vi "Lan07.vi"() -> ()   [LabVIEW 2022 SP3]
uses:
  StateMachineControl.ctl
  <vilib>/measure/NI_MAPro.lvlib
  <vilib>/measure/NI_MABase.lvlib
  <vilib>/measure/mascope.llb/Amplitude and Levels 1 chan.vi
panel:
  in  "Amplitude":dbl=1.0 format="%0.2p"
  out "High State Level":dbl format="%.2g"
  out "Pk-Pk Measured":dbl format="%.2p"
  out "Current State":T1
  in  "Stop":bool
  in  "Analyze Data":bool
  in  "Aquire Data":bool
  out "Waveform Graph":waveform(dbl)(graph)
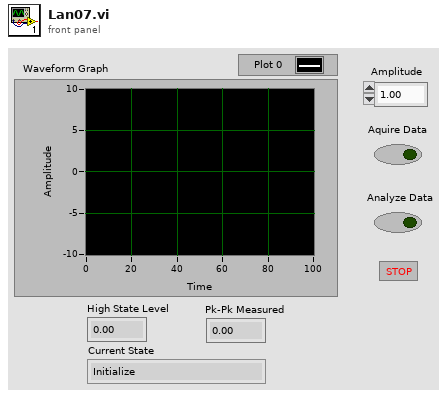
[diagram p1: front panel]
types:
  T1 = typedef "StateMachineControl.ctl" = enum16{"Initialize", "Stop", "Check for UI Events", "Aquire Data", "Analyze Data"}
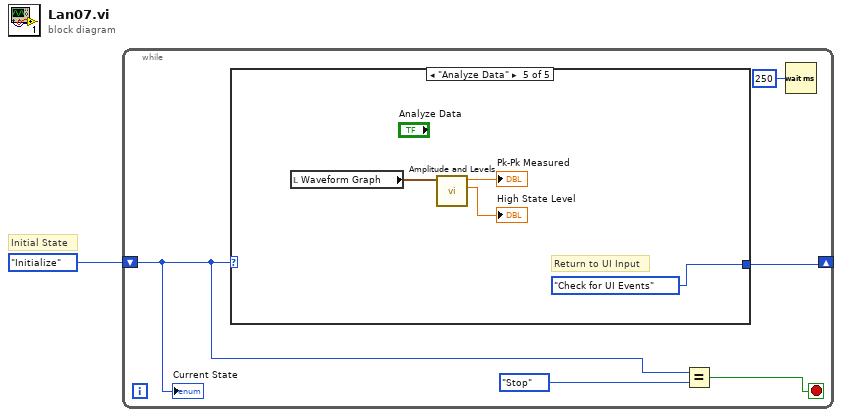
[diagram p0: block diagram]
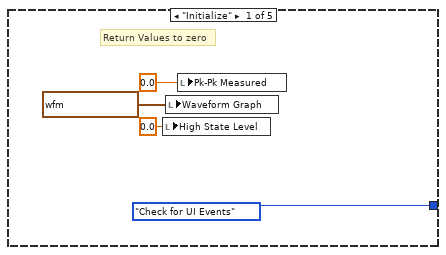
[diagram p2: hidden frame]
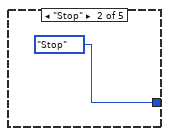
[diagram p3: hidden frame]
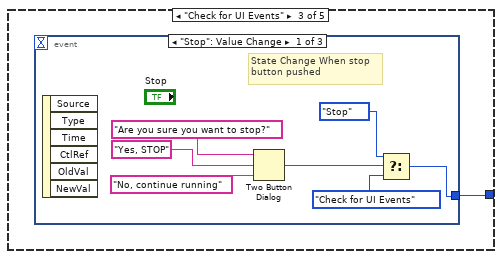
[diagram p4: hidden frame]
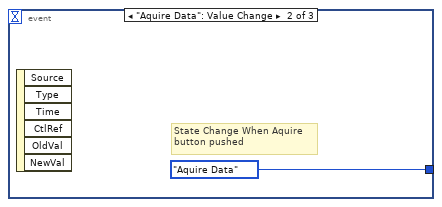
[diagram p5: hidden frame]
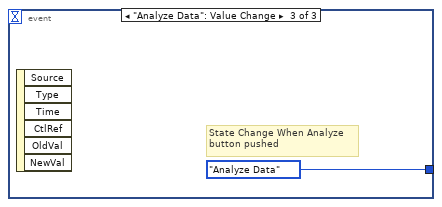
[diagram p6: hidden frame]
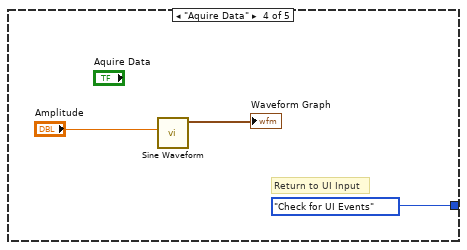
[diagram p7: hidden frame]
diagram:
  # "Initial State"
  n1 = while {
    shift-right: [w4] -> _
    shift-left: StateMachineControl."Initialize" -> [w2]
    stop <- w6 stop-if-true
    n2 = case shown="\"Analyze Data\"" w2 {
      tunnel: [StateMachineControl."Check for UI Events" StateMachineControl."Stop" w12 StateMachineControl."Check for UI Events" StateMachineControl."Check for UI Events"] -> w4
      frame "Initialize" {
        # "Return Values to zero"
        n3 = local write "High State Level"(0.0 ("high state level")) -> ()
        n4 = local write "Waveform Graph"(waveform(dbl) {"t0"=timestamp(0 s since 1904-01-01), "dt"=1.0, "Y"=[]} ("Waveform Graph")) -> ()
        n5 = local write "Pk-Pk Measured"(0.0 ("Amplitude Measured")) -> ()
      }
      frame "Stop" {
      }
      frame "Check for UI Events" {
        n6 = event shown="[0] \"Stop\": Value Change" {
          selector: _ -> [_ _ _]
          dyn-events: _ -> [_ _ _]
          timeout: _ -> [_ _ _]
          tunnel: [w13 StateMachineControl."Aquire Data" StateMachineControl."Analyze Data"] -> w12
          event "Stop": Value Change {
            # "State Change When stop\nbutton pushed"
            n7 = event-data() -> ()  [unwired: 1 in, 6 out]
            n8 = Two Button Dialog(message="Are you sure you want to stop?", 1:"No, continue running" ("Center Button Text (\"No\")"), 2:"Yes, STOP" ("Left Button Text (\"Yes\")")) -> (T button?=w14:bool)
            n9 = Select(t=StateMachineControl."Stop", s=w14, f=StateMachineControl."Check for UI Events") -> (s? t:f=w13:T1)
          }
          event "Aquire Data": Value Change {
            # "State Change When Aquire\nbutton pushed"
            n10 = event-data() -> ()  [unwired: 1 in, 6 out]
          }
          event "Analyze Data": Value Change {
            # "State Change When Analyze\nbutton pushed"
            n11 = event-data() -> ()  [unwired: 1 in, 6 out]
          }
        }
      }
      frame "Aquire Data" {
        # "Return to UI Input"
        n12 = call <vilib>:"Sine Waveform.vi"("amplitude"="Amplitude") -> ("signal out"=→"Waveform Graph":waveform(dbl))  [unwired: 9 in, 1 out]
      }
      frame "Analyze Data" {
        # "Return to UI Input"
        n13 = local read "Waveform Graph"() -> (w26:waveform(dbl))
        n14 = call-poly <vilib>:"Amplitude and Levels.vi"("signal in"=w26) -> ("high state level"=→"High State Level":dbl, "amplitude"=→"Pk-Pk Measured":dbl)  [unwired: 7 in, 2 out]
      }
    }
    n15 = Equal?(x=w2, y=StateMachineControl."Stop") -> (x = y?=w6:bool)
    n16 = Wait (ms)(milliseconds to wait=u32 250) -> ()  [unwired: 1 out]
    "Current State" <- w2
  }
